vi "Model IRF Fit Output String.vi"(5 "R^2":dbl, 7 "Reduced Chi^2":dbl, 8 "Error In":errorcluster, 9 "Delta Best Fit Parameters":dbl[](array[numeric]), 10 "Best Fit Parameters":dbl[](array[numeric]), 11 "Plot Name":string) -> (0 "Error Out":errorcluster, 3 "Fit Output Message":string)   [LabVIEW 2021, in "Fits.lvlib"]
uses:
  <vilib>/Utility/error.llb/Error Cluster From Error Code.vi
  <vilib>/ErrorRing/Error Ring.xnode
  Fits.lvlib
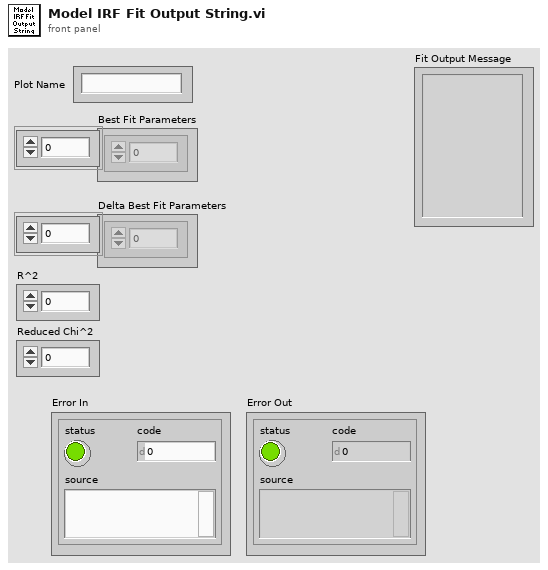
[diagram p1: front panel]
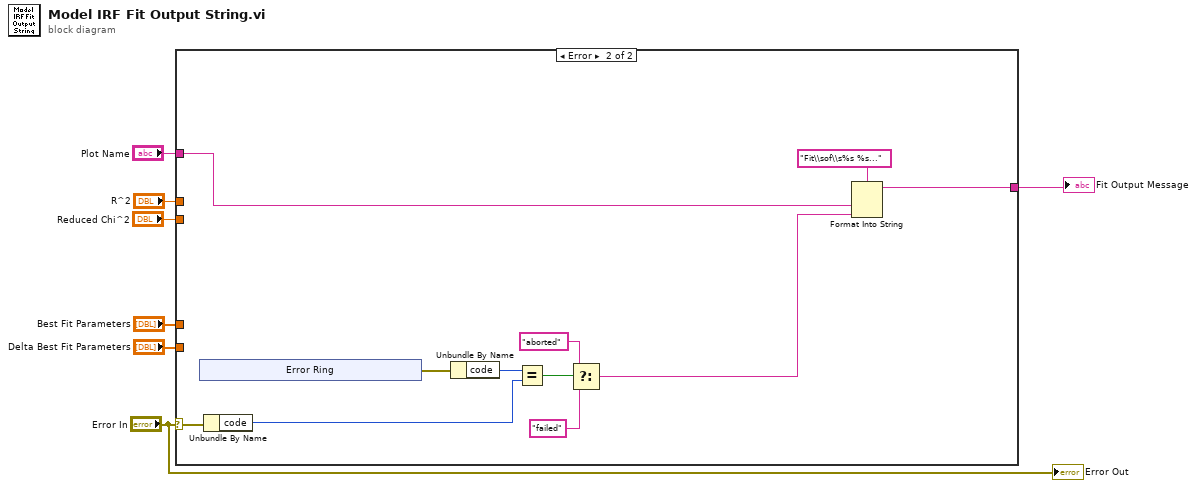
[diagram p0: block diagram]
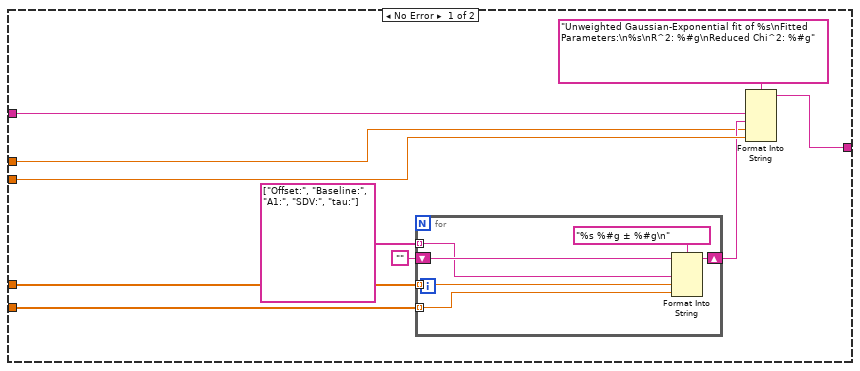
[diagram p2: hidden frame]
diagram:
  n1 = case shown="Error" "Error In" {
    selector: "Error In" -> [_ w29]
    tunnel: "Plot Name" -> [w10 w32]
    tunnel: "R^2" -> [w8 _]
    tunnel: "Best Fit Parameters" -> [w16 _]
    tunnel: "Delta Best Fit Parameters" -> [w15 _]
    tunnel: [w14 w34] -> w3
    tunnel: "Reduced Chi^2" -> [w12 _]
    frame No Error {
      n2 = for {
        tunnel: w16 -> [w20] mode=indexing
        tunnel: w15 -> [w19] mode=indexing
        tunnel: string[] ["Offset:", "Baseline:", "A1:", "SDV:", "tau:"] ("Parameter Names") -> [w21] mode=indexing
        shift-right: [w23] -> w9
        shift-left: "" -> [w22]
        n3 = Format Into String(format string="%s %#g ± %#g\n", initial string=w22, w21, w20, w19) -> (resulting string=w23:string)  [unwired: 1 in, 1 out]
      }
      n4 = Format Into String(format string="Unweighted Gaussian-Exponential fit of %s\nFitted Parameters:\n%s\nR^2: %#g\nReduced Chi^2: %#g", w10, w9, w8, w12) -> (resulting string=w14:string)  [unwired: 2 in, 1 out]
    }
    frame Error {
      n5 = xnode "Error Ring"() -> ("error out"=w31:errorcluster)
      n6 = Unbundle By Name(w29) -> ("code"=w28:i32)
      n7 = Unbundle By Name(w31) -> ("code"=w30:i32)
      n8 = Equal?(x=w30, y=w28) -> (x = y?=w27:bool)
      n9 = Select(t="aborted" ("input 4"), s=w27, f="failed" ("input 4")) -> (s? t:f=w24:string)
      n10 = Format Into String(format string="Fit\\sof\\s%s %s...", w32, w24) -> (resulting string=w34:string)  [unwired: 2 in, 1 out]
    }
  }
  "Fit Output Message" <- w3
  "Error Out" <- "Error In"
